vi "ZMQ Rep Test.vi"() -> ()   [LabVIEW 2019, in "RemoteControl.ZMQ.lvlib" / "RemoteControl.ZMQ.lvclass"]
uses:
  RemoteControl.ZMQ.lvclass
  C:/Program Files (x86)/National Instruments/LabVIEW 2019/user.lib/LevyLab/RemoteControl/RemoteControl/RemoteControl.lvclass
  <userlib>/LevyLab/RemoteControl/RemoteControl/RemoteControl.lvclass/RemoteControl.ctl
  <vilib>/addons/zeromq/zmq_context.lvclass
  <vilib>/addons/zeromq/socket_type.ctl
  <vilib>/addons/zeromq/zeromq.lvlib
  <vilib>/addons/zeromq/zmq_socket.lvclass
  <vilib>/addons/zeromq/socket_options.ctl
  <userlib>/LevyLab/RemoteControl/RemoteControl/RemoteControl.lvclass
  C:/Program Files (x86)/National Instruments/LabVIEW 2019/vi.lib/JKI/JKI SMO/SMO/SMO.lvclass
panel:
  out "error out":errorcluster
  in  "stop":bool
  out "Command":string
  out "ID":string
  out "Data":variant
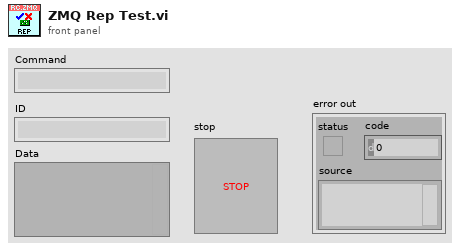
[diagram p1: front panel]
types:
  T1 = typedef "zeromq.lvlib/socket_options.ctl" = enum8{"NONE", "ZMQ_HWM", "<2>", "ZMQ_SWAP", "ZMQ_AFFINITY", "ZMQ_ROUTING_ID", "ZMQ_SUBSCRIBE", "ZMQ_UNSUBSCRIBE", "ZMQ_RATE", "ZMQ_RECOVERY_IVL", "ZMQ_MCAST_LOOP", "ZMQ_SNDBUF", "ZMQ_RCVBUF", "ZMQ_RCVMORE", "ZMQ_FD", "ZMQ_EVENTS", "ZMQ_TYPE", "ZMQ_LINGER", "ZMQ_RECONNECT_IVL", "ZMQ_BACKLOG", "ZMQ_RECOVERY_IVL_MSEC", "ZMQ_RECONNECT_IVL_MAX", "ZMQ_MAXMSGSIZE", "ZMQ_SNDHWM", "ZMQ_RCVHWM", "ZMQ_MULTICAST_HOPS", "<26>", "ZMQ_RCVTIMEO", "ZMQ_SNDTIMEO", "<29>", "<30>", "ZMQ_IPV4ONLY", "ZMQ_LAST_ENDPOINT", "ZMQ_ROUTER_MANDATORY", "ZMQ_TCP_KEEPALIVE", "ZMQ_TCP_KEEPALIVE_CNT", "ZMQ_TCP_KEEPALIVE_IDLE", "ZMQ_TCP_KEEPALIVE_INTVL", "ZMQ_TCP_ACCEPT_FILTER", "ZMQ_IMMEDIATE", "ZMQ_XPUB_VERBOSE", "ZMQ_ROUTER_RAW", "ZMQ_IPV6", "ZMQ_MECHANISM", "ZMQ_PLAIN_SERVER", "ZMQ_PLAIN_USERNAME", "ZMQ_PLAIN_PASSWORD", "ZMQ_CURVE_SERVER", "ZMQ_CURVE_PUBLICKEY", "ZMQ_CURVE_SECRETKEY", "ZMQ_CURVE_SERVERKEY", "ZMQ_PROBE_ROUTER", "ZMQ_REQ_CORRELATE", "ZMQ_REQ_RELAXED", "ZMQ_CONFLATE", "ZMQ_ZAP_DOMAIN", "ZMQ_ROUTER_HANDOVER", "ZMQ_TOS", "ZMQ_IPC_FILTER_PID", "ZMQ_IPC_FILTER_UID", "ZMQ_IPC_FILTER_GID", "ZMQ_CONNECT_ROUTING_ID", "ZMQ_GSSAPI_SERVER", "ZMQ_GSSAPI_PRINCIPAL", "ZMQ_GSSAPI_SERVICE_PRINCIPAL", "ZMQ_GSSAPI_PLAINTEXT", "ZMQ_HANDSHAKE_IVL", "<67>", "ZMQ_SOCKS_PROXY", "ZMQ_XPUB_NODROP", "ZMQ_BLOCKY", "ZMQ_XPUB_MANUAL", "ZMQ_XPUB_WELCOME_MSG", "ZMQ_STREAM_NOTIFY", "ZMQ_INVERT_MATCHING", "ZMQ_HEARTBEAT_IVL", "ZMQ_HEARTBEAT_TTL", "ZMQ_HEARTBEAT_TIMEOUT", "ZMQ_XPUB_VERBOSER", "ZMQ_CONNECT_TIMEOUT", "ZMQ_TCP_MAXRT", "ZMQ_THREAD_SAFE", "<82>", "<83>", "ZMQ_MULTICAST_MAXTPDU", "ZMQ_VMCI_BUFFER_SIZE", "ZMQ_VMCI_BUFFER_MIN_SIZE", "ZMQ_VMCI_BUFFER_MAX_SIZE", "ZMQ_VMCI_CONNECT_TIMEOUT", "ZMQ_USE_FD", "ZMQ_GSSAPI_PRINCIPAL_NAMETYPE", "ZMQ_GSSAPI_SERVICE_PRINCIPAL_NAMETYPE", "ZMQ_BINDTODEVICE", "ZMQ_ZAP_ENFORCE_DOMAIN", "ZMQ_LOOPBACK_FASTPATH", "ZMQ_METADATA", "ZMQ_MULTICAST_LOOP", "ZMQ_ROUTER_NOTIFY"}
  T2 = typedef "zeromq.lvlib/socket_type.ctl" = enum8{"ZMQ_PAIR", "ZMQ_PUB", "ZMQ_SUB", "ZMQ_REQ", "ZMQ_REP", "ZMQ_DEALER", "ZMQ_ROUTER", "ZMQ_PULL", "ZMQ_PUSH", "ZMQ_XPUB", "ZMQ_XSUB", "ZMQ_STREAM", "ZMQ_SERVER", "ZMQ_CLIENT", "ZMQ_RADIO", "ZMQ_DISH", "ZMQ_GATHER", "ZMQ_SCATTER", "ZMQ_DGRAM"}
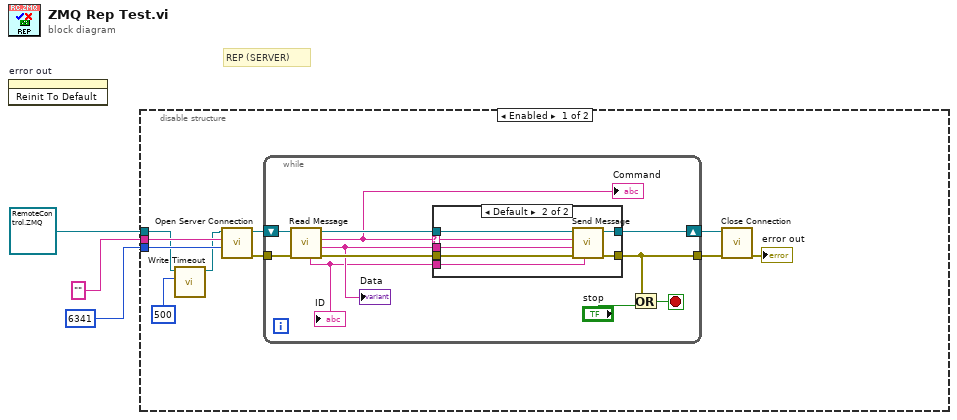
[diagram p0: block diagram]
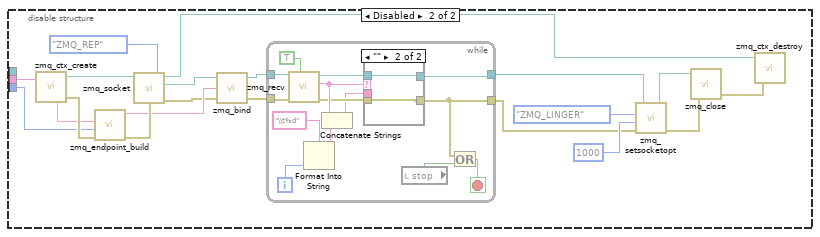
[diagram p3: hidden frame]
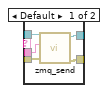
[diagram p4: hidden frame]
diagram:
  # "REP (SERVER)"
  n1 = invoke on="error out" class="Clust (strict)" method="Reinit To Default"() -> ()  [unwired: 3 in, 3 out]
  n2 = disable-structure shown="Enabled" {
    disable-tunnel: refnum<class "RemoteControl.ZMQ.lvclass"> refnum ("RemoteControl.ZMQ.lvlib:RemoteControl.ZMQ.lvclass") -> [w6 _]
    disable-tunnel: u16 6341 ("Port") -> [w9 w41]
    disable-tunnel: "" ("Address") -> [w8 w40]
    frame Enabled {
      n3 = call <userlib>:"Write Timeout.vi"("timeout (ms) [500]"=500 ("timeout in ms (100)"), "RemoteControl in"=w6) -> ("RemoteControl out"=w5:refnum<class "RemoteControl.ZMQ.lvclass">)  [unwired: 8 in, 1 out]
      n4 = call-dynamic "Open Server Connection.vi"("port"=w9, "address"=w8, "RemoteControl.ZMQ in"=w5) -> ("error out"=w12:errorcluster, "RemoteControl.ZMQ out"=w13:refnum<class "RemoteControl.ZMQ.lvclass">)  [unwired: 7 in]
      n5 = while {
        tunnel: w12 -> [w23]
        tunnel: [w19] -> w10
        shift-right: [w20] -> w11
        shift-left: w13 -> [w24]
        stop <- w18 stop-if-true
        n6 = call-dynamic "Read Message.vi"("error in (no error)"=w23, "RemoteControl.ZMQ in"=w24) -> ("error out"=w22:errorcluster, "Data"=w15:string, "Command"=w16:string, "RemoteControl.ZMQ out"=w21:refnum<class "RemoteControl.ZMQ.lvclass">, "ID"=w14:string)  [unwired: 5 in]
        "Data" <- w15
        "ID" <- w14
        "Command" <- w16
        n7 = case shown="Default" w16 {
          selector: w16 -> [_ w28]
          tunnel: w22 -> [w25 w33]
          tunnel: w21 -> [w26 w32]
          tunnel: [w26 w31] -> w20
          tunnel: [w25 w30] -> w19
          tunnel: w14 -> [_ w29]
          tunnel: w15 -> [_ w27]
          frame "" {
            # "no incoming msg:\ndo nothing"
          }
          frame Default {
            n8 = call-dynamic "Send Message.vi"("ID"=w29, "error in (no error)"=w33, "Data"=w27, "Command"=w28, "RemoteControl.ZMQ in"=w32) -> ("error out"=w30:errorcluster, "RemoteControl.ZMQ out"=w31:refnum<class "RemoteControl.ZMQ.lvclass">)  [unwired: 5 in]
          }
        }
        n9 = Or(x=w19, y="stop") -> (x .or. y?=w18:bool)
      }
      n10 = call-dynamic "Close Connection.vi"("error in (no error)"=w10, "RemoteControl.ZMQ in"=w11) -> ("error out"=→"error out":errorcluster)  [unwired: 8 in, 1 out]
    }
    frame Disabled {
      n11 = call <vilib>:"zmq_ctx_create.vi"() -> ("error out"=w50:errorcluster, "context out"=w52:refnum<class "zmq_context.lvclass">)  [unwired: 4 in]
      n12 = call <vilib>:"zmq_endpoint_build.vi"("error in"=w50, "port"=w41, "address"=w40) -> ("error out"=w49:errorcluster, "endpoint"=w38:string)  [unwired: 2 in, 1 out]
      n13 = call <vilib>:"zmq_socket.vi"("error in"=w49, "socket type"=socket_type."ZMQ_REP", "context in"=w52) -> ("error out"=w37:errorcluster, "socket out"=w39:refnum<class "zmq_socket.lvclass">, "context out"=w42:refnum<class "zmq_context.lvclass">)  [unwired: 2 in]
      n14 = call <vilib>:"zmq_bind.vi"("error in"=w37, "endpoint"=w38, "socket in"=w39) -> ("error out"=w35:errorcluster, "socket out"=w36:refnum<class "zmq_socket.lvclass">)  [unwired: 1 in]
      n15 = while {
        tunnel: w35 -> [w63]
        tunnel: w36 -> [w64]
        tunnel: [w61] -> w45
        tunnel: [w56] -> w34
        i -> [w59]
        stop <- w65 stop-if-true
        n16 = call <vilib>:"zmq_recv.vi"("no block? (F)"=TRUE, "error in"=w63, "socket in"=w64) -> ("error out"=w54:errorcluster, "data"=w55:string, "socket out"=w62:refnum<class "zmq_socket.lvclass">)  [unwired: 2 in, 2 out]
        n17 = Format Into String(format string="\\t%d" ("Command"), w59) -> (resulting string=w58:string)  [unwired: 2 in, 1 out]
        n18 = Concatenate Strings(w55, w58) -> (w53:string)
        n19 = case shown="\"\"" w55 {
          tunnel: w62 -> [w71 w73]
          tunnel: [w70 w73] -> w61
          tunnel: [w69 w72] -> w56
          tunnel: w54 -> [w67 w72]
          tunnel: w53 -> [w68 _]
          frame Default {
            n20 = call <vilib>:"zmq_send.vi"("error in"=w67, "data"=w68, "socket in"=w71) -> ("error out"=w69:errorcluster, "socket out"=w70:refnum<class "zmq_socket.lvclass">)  [unwired: 4 in]
          }
          frame "" {
          }
        }
        n21 = local read "stop"() -> (w66:bool)
        n22 = Or(x=w56, y=w66) -> (x .or. y?=w65:bool)
      }
      n23 = call <vilib>:"zmq_setsocketopt.vi"("error in"=w34, "value"=1000, "option"=socket_options."ZMQ_LINGER", "socket in"=w45) -> ("error out"=w44:errorcluster, "socket out"=w46:refnum<class "zmq_socket.lvclass">)  [unwired: 2 in]
      n24 = call <vilib>:"zmq_close.vi"("error in"=w44, "socket"=w46) -> ("error out"=w43:errorcluster)  [unwired: 3 in]
      n25 = call <vilib>:"zmq_ctx_destroy.vi"("error in"=w43, "context in"=w42) -> ()  [unwired: 3 in, 1 out]
    }
  }
